vi "Current Date and Time.vi"() -> (0 "Current Time":string, 1 "Current Date":string)   [LabVIEW 2018, in "ASI TG-1000.lvlib"]
uses:
  ASI TG-1000.lvlib
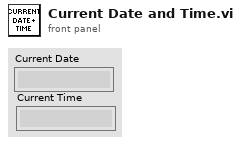
[diagram p1: front panel]
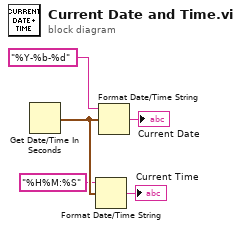
[diagram p0: block diagram]
diagram:
  n1 = Get Date/Time In Seconds() -> (seconds since 1Jan1904=w4:timestamp)
  n2 = Format Date/Time String(time format string (%c)="%H%M:%S", seconds (now)=w4) -> (date/time string=→"Current Time":string)  [unwired: 1 in]
  n3 = Format Date/Time String(time format string (%c)="%Y-%b-%d", seconds (now)=w4) -> (date/time string=→"Current Date":string)  [unwired: 1 in]
